vi "NewTestRole.vi"(10 "NewTestRole.lvclass 2":refnum<class "NewTestRole.lvclass">, 11 "Game in":refnum<class "Game.lvclass">) -> (0 "Game out":refnum<class "Game.lvclass">, 2 "Robot out":refnum<class "Robot.lvclass">, 3 "NewTestRole.lvclass":refnum<class "NewTestRole.lvclass">)   [LabVIEW 2022 SP3, in "NewTestRole.lvclass"]
uses:
  NewTestRole.lvclass
  Robot_class/Robot.lvclass
  Game_class/Game.lvclass
  C:/Users/ebert/Documents/codes/ssl/ssl/SSL_AI/Role_class/Role.lvclass
  Role_class/Role.lvclass/Role.ctl
  NewTestTactic_class/Control 1.ctl
  Role_class/Read Tacticbook.vi
  Role_class/Read tactic_index.vi
  Role_class/Write Tacticbook.vi
  Role_class/Write tactic_index.vi
  Role_class/Read RobotRef.vi
  Tacticbook_class/Tacticbook.lvclass
  NewTestTactic_class/NewTestTactic.lvclass
panel:
  out "error out":errorcluster
  in  "error in (no error)":errorcluster
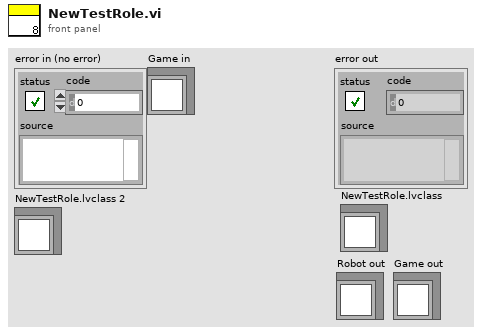
[diagram p1: front panel]
types:
  T1 = typedef "Control 1.ctl" = enum16{"ebo1", "ebo2", "bo3"}
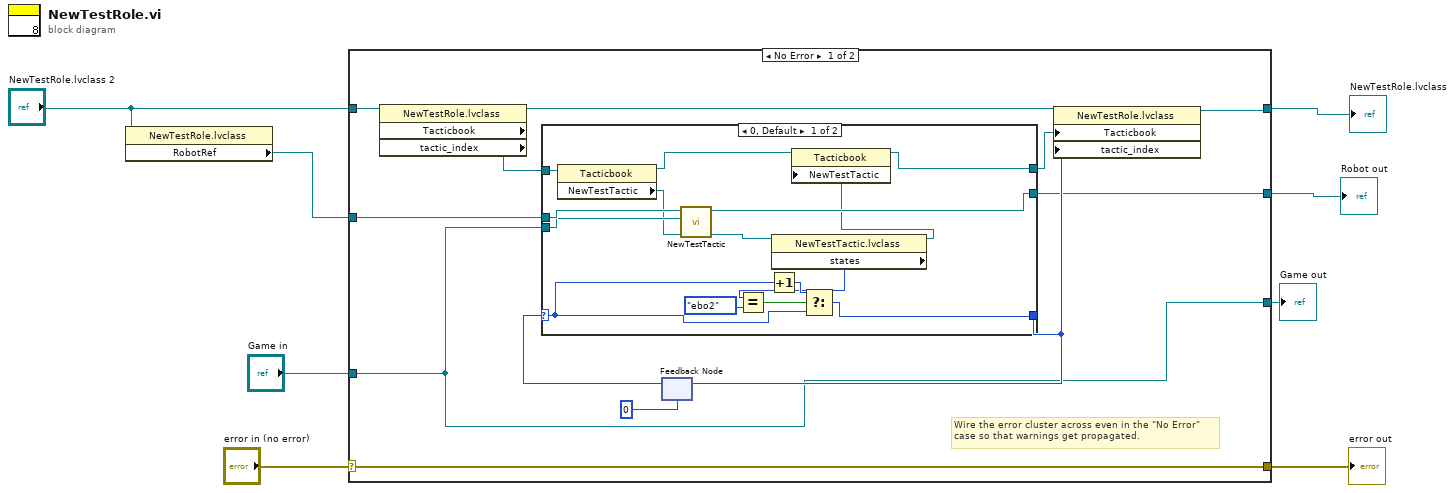
[diagram p0: block diagram]
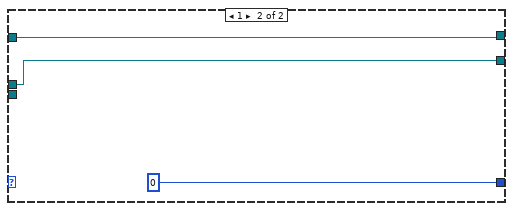
[diagram p2: hidden frame]
diagram:
  n1 = property class="NewTestRole.lvclass"(reference="NewTestRole.lvclass 2") -> ("RobotRef"=w3:refnum<class "Robot.lvclass">)  [unwired: 1 in, 2 out]
  n2 = case shown="No Error" "error in (no error)" {
    selector: "error in (no error)" -> [w20 w42]
    tunnel: [w20 w42] -> w7
    tunnel: [w18 w41] -> w2
    tunnel: "NewTestRole.lvclass 2" -> [w19 w41]
    tunnel: w3 -> [w12 w40]
    tunnel: [w11 w40] -> w6
    tunnel: [w9 w39] -> w5
    tunnel: "Game in" -> [w9 w39]
    frame No Error {
      # "Wire the error cluster across even in the \"No Error\"\ncase so that warnings get propagated."
      n3 = property class="NewTestRole.lvclass" props=["Tacticbook", "tactic_index"](reference=w19) -> (reference out=w17:refnum<class "NewTestRole.lvclass">, "Tacticbook"=w14:refnum<class "Tacticbook.lvclass">)  [unwired: 1 in, 2 out]
      n4 = feedback #1(0) -> (w15:i32)
      n5 = case shown="0, Default" w15 {
        selector: w15 -> [w32 _]
        tunnel: [w33 0] -> w13
        tunnel: w14 -> [w35 w36]
        tunnel: w12 -> [w28 w38]
        tunnel: [w25 w38] -> w11
        tunnel: [w29 w36] -> w10
        tunnel: w9 -> [w27 _]
        frame 0, Default {
          n6 = property class="Tacticbook"(reference=w35) -> (reference out=w30:refnum<class "Tacticbook.lvclass">, "NewTestTactic"=w26:refnum<class "NewTestTactic.lvclass">)  [unwired: 1 in, 1 out]
          n7 = call "NewTestTactic.vi"("NewTestTactic.lvclass"=w26, "Game in"=w27, "Robot"=w28) -> ("NewTestTactic.lvclass 2"=w23:refnum<class "NewTestTactic.lvclass">, "Robot out"=w25:refnum<class "Robot.lvclass">)  [unwired: 7 in]
          n8 = Increment(x=w32) -> (x+1=w31:i32)
          n9 = property class="NewTestTactic.lvclass"(reference=w23) -> (reference out=w24:refnum<class "NewTestTactic.lvclass">, "states"=w22:T1)  [unwired: 1 in, 1 out]
          n10 = Equal?(x=w22, y=Control_1."ebo2") -> (x = y?=w34:bool)
          n11 = property class="Tacticbook"(reference=w30, "NewTestTactic"=w24) -> (reference out=w29:refnum<class "Tacticbook.lvclass">)  [unwired: 1 in, 1 out]
          n12 = Select(t=w31, s=w34, f=w32) -> (s? t:f=w33:i32)
        }
        frame 1 {
        }
      }
      n13 = feedback-in #1(w13) -> ()
      n14 = property class="NewTestRole.lvclass"(reference=w17, "Tacticbook"=w10, "tactic_index"=w13) -> (reference out=w18:refnum<class "NewTestRole.lvclass">)  [unwired: 1 in, 1 out]
    }
    frame Error {
    }
  }
  "error out" <- w7
  "Robot out" <- w6
  "Game out" <- w5
  "NewTestRole.lvclass" <- w2
